vi "Configure Modulation (PM).vi"(0 "VISA resource name":refnum<visa-resource-name>, 1 "Enable Phase Modulation (T:Enable)":bool=TRUE, 2 "Modulation Waveform (0: Sine)":u16(ring) items=["Sine", "Square", "Triangle", "UpRamp", "DnRamp", "Noise", "Arb"], 5 "PM Source (0: Internal)":u16(ring) items=["Internal", "External"], 7 "Channel (1:Channel 1)":i32(ring)=1 items=["Channel 1"=1, "Channel 2"=2], 9 "Phase Deviation (0.0 degree)":dbl min=0.0 max=360.0 format="%.1f", 11 "error in (no error)":errorcluster, 12 "Modulation Frequency (100 Hz)":dbl=100.0) -> (4 "VISA resource name out":refnum<visa-resource-name>, 15 "error out":errorcluster)   [LabVIEW 2023, in "Siglent SDG X Series.lvlib"]
doc: "Configures and enables phase modulation (PM). In PM, the amplitude of the carrier is varied by the amplitude of the modulating waveform. \n\n<B>Note:</B> The carrier waveform shape and parameters are set by the Configure Standard Waveform VI."
uses:
  Siglent SDG X Series.lvlib
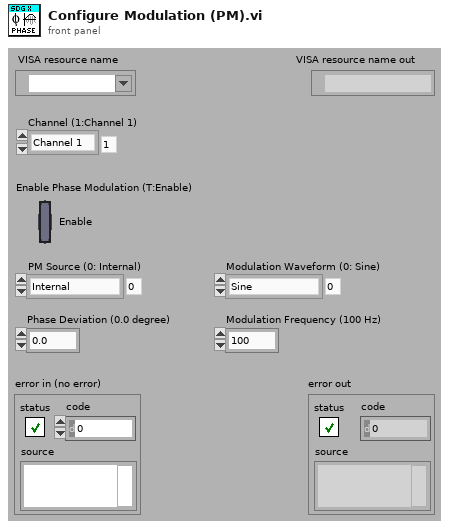
[diagram p1: front panel]
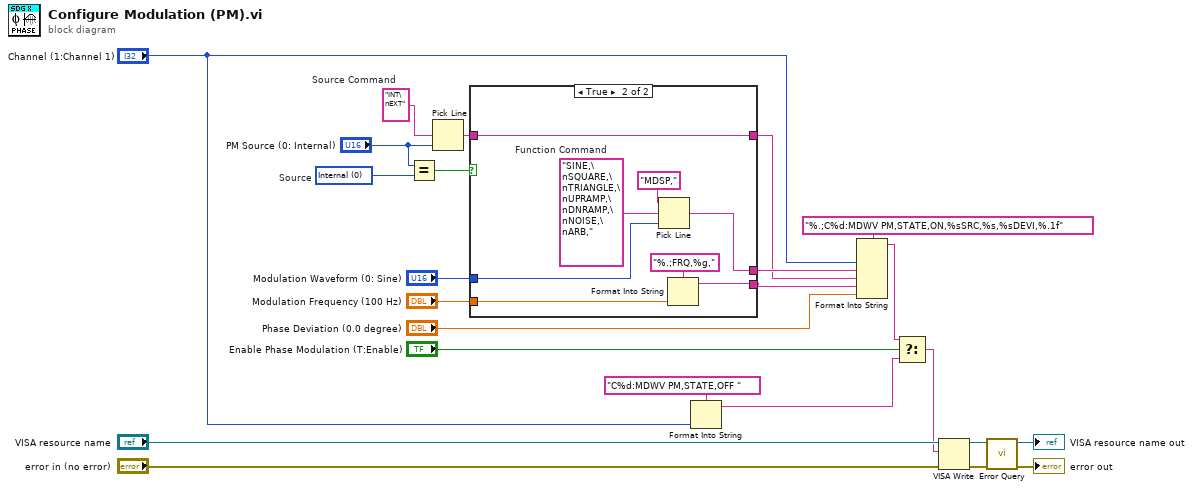
[diagram p0: block diagram]
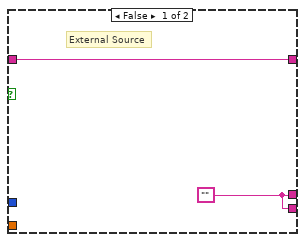
[diagram p2: hidden frame]
diagram:
  w13 = u16 0 items=["Internal", "External"]  # Source
  w14 = "INT\nEXT"  # Source Command
  n1 = Equal?(x="PM Source (0: Internal)", y=w13) -> (x = y?=w12:bool)
  n2 = Pick Line(multi-line string=w14, line index="PM Source (0: Internal)") -> (output string=w11:string)  [unwired: 1 in]
  n3 = case shown="True" w12 {
    tunnel: w11 -> [w26 w32]
    tunnel: "Modulation Waveform (0: Sine)" -> [_ w33]
    tunnel: "Modulation Frequency (100 Hz)" -> [_ w29]
    tunnel: [w26 w32] -> w8
    tunnel: [w25 w30] -> w9
    tunnel: [w25 w27] -> w7
    frame False {
      w25 = ""
      # "External Source"
    }
    frame True {
      w34 = "SINE,\nSQUARE,\nTRIANGLE,\nUPRAMP,\nDNRAMP,\nNOISE,\nARB,"  # Function Command
      n4 = Pick Line(string ("")="MDSP,", multi-line string=w34, line index=w33) -> (output string=w30:string)
      n5 = Format Into String(format string="%.;FRQ,%g,", w29) -> (resulting string=w27:string)  [unwired: 2 in, 1 out]
    }
  }
  n6 = Format Into String(format string="C%d:MDWV PM,STATE,OFF ", "Channel (1:Channel 1)") -> (resulting string=w3:string)  [unwired: 2 in, 1 out]
  n7 = Format Into String(format string="%.;C%d:MDWV PM,STATE,ON,%sSRC,%s,%sDEVI,%.1f", "Channel (1:Channel 1)", w9, w8, w7, "Phase Deviation (0.0 degree)") -> (resulting string=w4:string)  [unwired: 2 in, 1 out]
  n8 = Select(t=w4, s="Enable Phase Modulation (T:Enable)", f=w3) -> (s? t:f=w2:string)
  n9 = VISA Write(VISA resource name="VISA resource name", write buffer=w2, error in (no error)="error in (no error)") -> (VISA resource name out=w22:refnum<visa-resource-name>, error out=w21:errorcluster)  [unwired: 1 out]
  n10 = call "Error Query.vi"("error in (no error)"=w21, "VISA resource name"=w22) -> ("error out"=→"error out":errorcluster, "VISA resource name out"=→"VISA resource name out":refnum<visa-resource-name>)  [unwired: 6 in, 2 out]
